vi "GetAttribute.vi"(0 "reference in":refnum<class "G#BaseClass2.lvclass">, 5 "error in (no error)":errorcluster) -> (12 "Locked":bool, 14 "reference out":refnum<class "G#BaseClass2.lvclass">, 16 "Numeric":dbl, 17 "Array":dbl[](array[numeric]), 19 "error out":errorcluster)   [LabVIEW 2017, in "G#BaseClass2.lvclass"]
uses:
  G#BaseClass2.lvclass
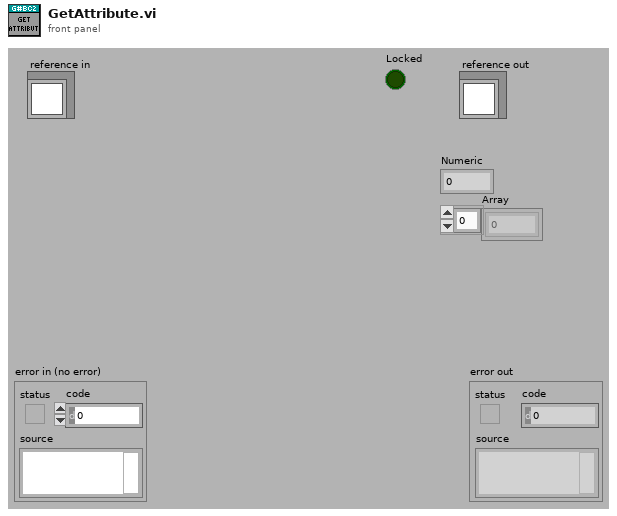
[diagram p1: front panel]
types:
  T1 = typedef "G#BaseClass2.lvclass/ObjectAttributes.ctl" = cluster{"Numeric":dbl, "Array":dbl[]}
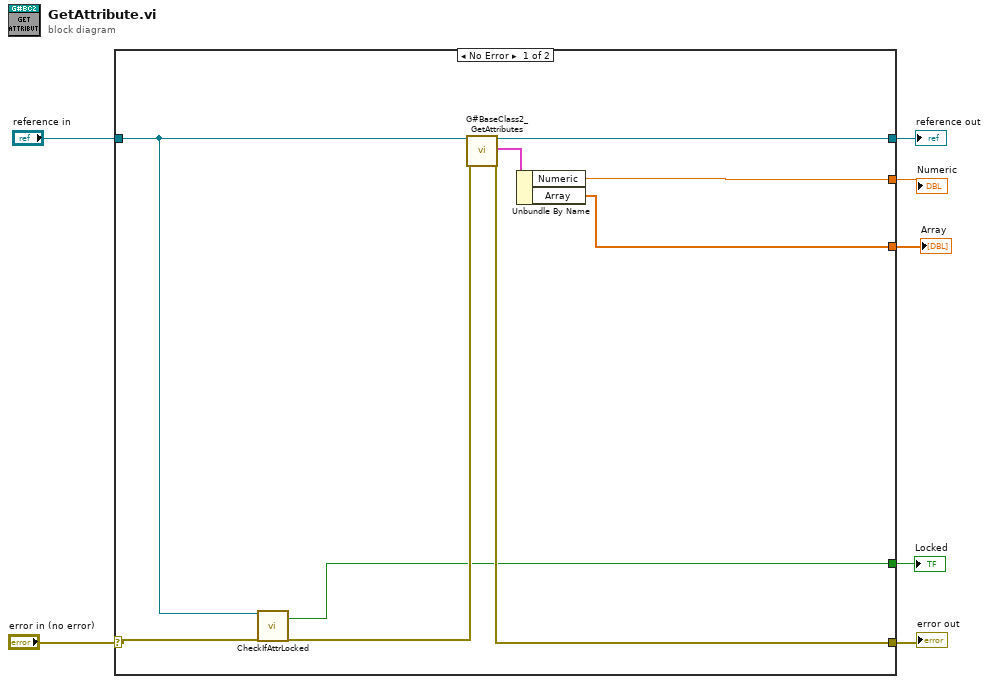
[diagram p0: block diagram]
diagram:
  n1 = case shown="No Error" "error in (no error)" {
    selector: "error in (no error)" -> [w11 w18]
    tunnel: [w15 w18] -> w6
    tunnel: [w14 w17] -> w4
    tunnel: "reference in" -> [w10 w17]
    tunnel: [w13 _] -> w3
    tunnel: [w12 _] -> w2
    tunnel: [w8 _] -> w1
    frame No Error {
      n2 = call-dynamic "CheckIfAttrLocked.vi"("reference in"=w10, "error in (no error)"=w11) -> ("locked"=w8:bool, "error out"=w9:errorcluster)  [unwired: 15 in, 1 out]
      n3 = call "G#BaseClass2_GetAttributes.vi"("reference in"=w10, "error in (no error)"=w9) -> ("reference out"=w14:refnum<class "G#BaseClass2.lvclass">, "attributes"=w16:T1, "error out"=w15:errorcluster)  [unwired: 14 in, 1 out]
      n4 = Unbundle By Name(w16) -> ("Numeric"=w13:dbl, "Array"=w12:dbl[])
    }
    frame Error {
    }
  }
  "error out" <- w6
  "reference out" <- w4
  "Numeric" <- w3
  "Array" <- w2
  "Locked" <- w1
